vi "Local run of Caraya test.vi"() -> ()   [LabVIEW 2020]
uses:
  Class/Caraya Unit Test/Caraya Unit Test.lvclass
  Class/Action/Project Action/Project Action.lvclass
  C:/Current projects/WS/LV32.2020..ProjectBuilder/Class/Action/Project Action/Project Action.lvclass
  C:/Current projects/WS/LV32.2020..ProjectBuilder/Interface/Action Interface/Action Interface.lvclass
  C:/Current projects/WS/LV32.2020..ProjectBuilder/Class/Caraya Unit Test/Caraya Unit Test.lvclass
panel:
  out "Success?":bool
  out "error out":errorcluster
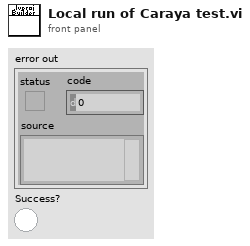
[diagram p1: front panel]
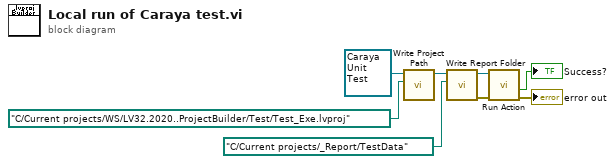
[diagram p0: block diagram]
diagram:
  n1 = call "Write Project Path.vi"("Project Path"=path "C:/Current projects/WS/LV32.2020..ProjectBuilder/Test/Test_Exe.lvproj", "Project Action in"=refnum<class "Caraya Unit Test.lvclass"> refnum ("ProjectBuilder.lvlib:Caraya Unit Test.lvclass")) -> ("Project Action out"=w7:refnum<class "Caraya Unit Test.lvclass">)  [unwired: 8 in, 1 out]
  n2 = call "Write Report Folder.vi"("Report Folder"=path "C:/Current projects/_Report/TestData", "Project Action in"=w7) -> ("error out"=w3:errorcluster, "Project Action out"=w4:refnum<class "Caraya Unit Test.lvclass">)  [unwired: 8 in]
  n3 = call "Run Action.vi"("error in (no error)"=w3, "Project Action"=w4) -> ("error out"=→"error out":errorcluster, "Success?"=→"Success?":bool)  [unwired: 7 in, 1 out]
